vi "Treatment.vi"(8 "error in (no error)":errorcluster caption="entrée d'erreur (pas d'erreur)", 11 "Load_Diabetes en entrée":refnum<class "Load_Diabetes.lvclass">) -> (0 "error out":errorcluster caption="sortie d'erreur", 2 "Tableau":string[][](array[string]), 3 "Load_Diabetes en sortie":refnum<class "Load_Diabetes.lvclass">)   [LabVIEW 2020, in "Load_Diabetes.lvclass"]
uses:
  Load_Diabetes.lvclass
  Load_Diabetes.lvclass/Load_Diabetes.ctl
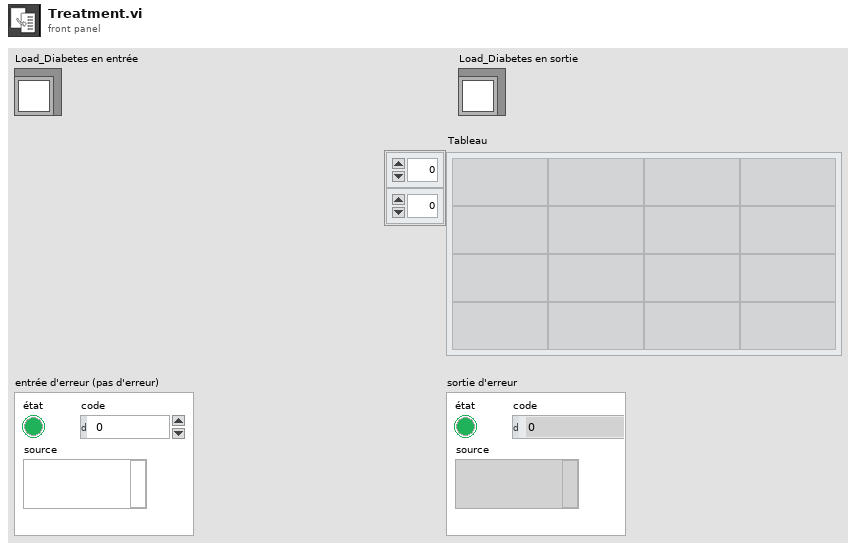
[diagram p1: front panel]
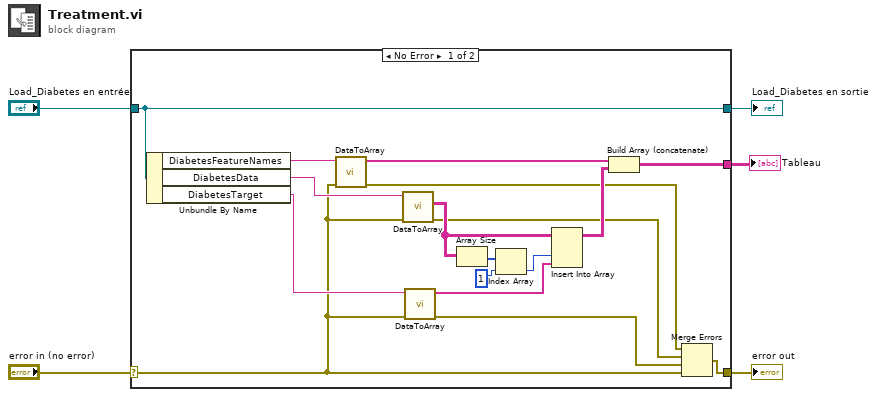
[diagram p0: block diagram]
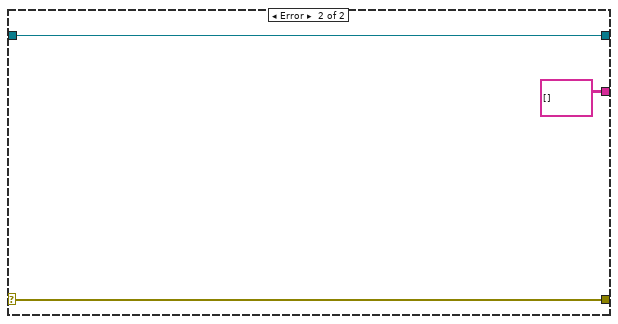
[diagram p2: hidden frame]
diagram:
  n1 = case shown="No Error" "error in (no error)" {
    selector: "error in (no error)" -> [w8 w25]
    tunnel: [w16 w25] -> w4
    tunnel: [w18 w24] -> w2
    tunnel: "Load_Diabetes en entrée" -> [w18 w24]
    tunnel: [w17 string[][] []] -> w1
    frame No Error {
      n2 = Unbundle By Name(w18) -> ("DiabetesFeatureNames"=w15:string, "DiabetesData"=w12:string, "DiabetesTarget"=w9:string)
      n3 = call "DataToArray.vi"("sortie d'erreur"=w8, "Return value"=w15) -> ("sortie d'erreur"=w14:errorcluster, "String 1DArray"=w13:string[])  [unwired: 6 in, 2 out]
      n4 = call "DataToArray.vi"("sortie d'erreur"=w8, "Return value"=w12) -> ("sortie d'erreur"=w10:errorcluster, "String 2DArray"=w11:string[][])  [unwired: 6 in, 2 out]
      n5 = call "DataToArray.vi"("sortie d'erreur"=w8, "Return value"=w9) -> ("sortie d'erreur"=w7:errorcluster, "String 1DArray"=w6:string[])  [unwired: 6 in, 2 out]
      n6 = Array Size(array=w11) -> (size(s)=w20:i32[])
      n7 = Index Array(array=w20, index=1 ("indice")) -> (element=w19:i32)
      n8 = Insert Into Array(array=w11, index (col)=w19, new element=w6) -> (w21:string[][])  [unwired: 1 in]
      n9 = Build Array (concatenate)(w13, w21) -> (w17:string[][])
      n10 = Merge Errors(w14, w10, w7, w8) -> (w16:errorcluster)
    }
    frame Error {
    }
  }
  "error out" <- w4
  "Load_Diabetes en sortie" <- w2
  "Tableau" <- w1
